vi "PRM - GetParameter.vi"(8 "error in (no error)":errorcluster, 11 "PRM":T1) -> (0 "error out":errorcluster, 3 "PRM OUT":T1, 5 "ParameterString":string)   [LabVIEW 2015]
doc: "Low Level function call. Converts LabVIEW enumeration to xiAPI parameter String."
uses:
  C:/GIT/Cameras3.x/Integrations/Labview/xiLib/xiLIB_32bit/xiLIB/xiCamLib/API/x86/xiApi.NET.dll
  xiLIB_32bit/xiLIB/xiCamLib/API/x86/xiApi.NET.dll
  PRM_v2.ctl
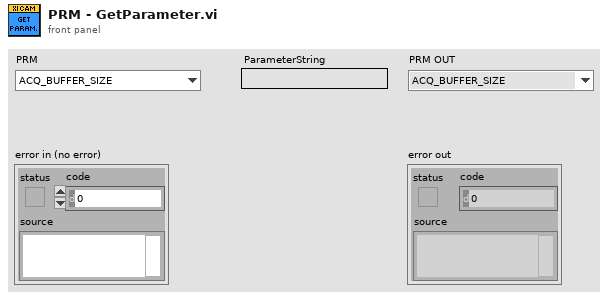
[diagram p1: front panel]
types:
  T1 = typedef "PRM_v2.ctl" = enum16{"ACQ_BUFFER_SIZE", "ACQ_FRAME_BURST_COUNT", "ACQ_TIMING_MODE", "ACQ_TRANSPORT_BUFFER_SIZE", "AE_MAX_LIMIT", "AEAG", "AEAG_LEVEL", "API_VERSION", "AG_MAX_LIMIT", "APPLY_CMS", "AUTO_BANDWIDTH_CALCULATION", "AUTO_WB", "AVAILABLE_BANDWIDTH", "AVAILABLE_BANDWIDTH_MAX", "AVAILABLE_BANDWIDTH_MIN", "BPC", "BUFFER_POLICY", "BUFFERS_QUEUE_SIZE", "CC_MATRIX_00", "CC_MATRIX_01", "CC_MATRIX_02", "CC_MATRIX_03", "CC_MATRIX_10", "CC_MATRIX_11", "CC_MATRIX_12", "CC_MATRIX_13", "CC_MATRIX_20", "CC_MATRIX_21", "CC_MATRIX_22", "CC_MATRIX_23", "CC_MATRIX_30", "CC_MATRIX_31", "CC_MATRIX_32", "CC_MATRIX_33", "CHIP_TEMP", "CMS", "COLOR_FILTER_ARRAY", "COOLING", "DEBOUNCE_EN", "DEBOUNCE_POL", "DEBOUNCE_T0", "DEBOUNCE_T1", "DEBUG_LEVEL", "DEFAULT_CC_MATRIX", "DEVICE_INSTANCE_PATH", "DEVICE_MODEL_ID", "DEVICE_NAME", "DEVICE_SN", "DEVICE_TYPE", "DEVICE_USER_ID", "DOWNSAMPLING", "DOWNSAMPLING_MAX", "DOWNSAMPLING_MIN", "DOWNSAMPLING_TYPE", "DRV_VERSION", "EXP_PRIORITY", "EXPOSURE", "EXPOSURE_DIRECT_UPDATE", "EXPOSURE_MAX", "EXPOSURE_MIN", "FFS_FILE_NAME", "FPGA1_VERSION", "FRAMERATE", "FRAMERATE_MAX", "FRAMERATE_MIN", "FREE_FFS_SIZE", "GAIN", "GAIN_DIRECT_UPDATE", "GAIN_MAX", "GAIN_MIN", "GAMMAC", "GAMMAY", "GPI_LEVEL", "GPI_MODE", "GPI_SELECTOR", "GPI_SELECTOR_MAX", "GPI_SELECTOR_MIN", "GPO_MODE", "GPO_SELECTOR", "GPO_SELECTOR_MAX", "GPO_SELECTOR_MIN", "HDR", "HDR_T1", "HDR_T2", "HEIGHT", "HEIGHT_MAX", "HEIGHT_MIN", "HOUSE_TEMP", "IMAGE_DATA_FORMAT", "IMAGE_IS_COLOR", "INPUT_CMS_PROFILE", "IS_COOLED", "IS_DEVICE_EXIST", "KNEEPOINT1", "KNEEPOINT2", "LED_MODE", "LED_SELECTOR", "LED_SELECTOR_MAX", "LED_SELECTOR_MIN", "LIMIT_BANDWIDTH", "LIMIT_BANDWIDTH_MAX", "LIMIT_BANDWIDTH_MIN", "LUT_EN", "LUT_INDEX", "LUT_INDEX_MAX", "LUT_INDEX_MIN", "LUT_VALUE", "LUT_VALUE_MAX", "LUT_VALUE_MIN", "MANUAL_WB", "MCU1_VERSION", "MCU2_VERSION", "OFFSET_X", "OFFSET_X_MAX", "OFFSET_X_MIN", "OFFSET_Y", "OFFSET_Y_MAX", "OFFSET_Y_MIN", "OUTPUT_CMS_PROFILE", "OUTPUT_DATA_BIT_DEPTH", "OUTPUT_DATA_PACKING", "READ_FILE_FFS", "RECENT_FRAME", "SENSOR_DATA_BIT_DEPTH", "SENSOR_MODE", "SENSOR_TAPS", "SHARPNESS", "SHUTTER_TYPE", "TARGET_TEMP", "TRG_DELAY", "TRG_SELECTOR", "TRG_SOFTWARE", "TRG_SOURCE", "USED_FFS_SIZE", "WB_KB", "WB_KG", "WB_KR", "WIDTH", "WIDTH_MAX", "WIDTH_MIN", "WRITE_FILE_FFS", "ACQ_BUFFER_SIZE_UNIT", "ACQ_TRANSPORT_BUFFER_COMMIT", "AEAG_ROI_HEIGHT", "AEAG_ROI_OFFSET_X", "AEAG_ROU_OFFSET_Y", "AEAG_ROI_WIDTH", "API_CONTEXT_LIST", "BINNING_HORIZONTAL", "BINNING_SELECTOR", "BINNING_VERTICAL", "COLUMN_FPN_CORRECTION", "COUNTER_SELECTOR", "COUNTER_VALUE", "DECIMATION_HORIZONTAL", "DECIMATION_SELECTOR", "DECIMATION_VERTICAL", "DEVICE_ID", "DEVICE_LOCATION_PATH", "DEVICE_MANIFEST", "DEVICE_RESET", "DEVICE_SENS_SN", "EXPOSURE_BURST_COUNT", "FFS_ACCESS_KEY", "GAIN_SELECTOR", "HW_REVISION", "IMAGE_BLACK_LEVEL", "IMAGE_DATA_BIT_DEPTH", "IMAGE_DATA_FORMAT_RGB32_ALPHA", "IMAGE_PAYLOAD_SIZE", "LENS_APERTURE_VALUE", "LENS_FEATURE", "LENS_FEATURE_SELECTOR", "LENS_FOCAL_LENGTH", "LENS_FOCUS_DISTANCE", "LENS_FOCUS_MOVE", "LENS_FOCUS_MOVEMENT_VALUE", "LENS_MODE", "OUTPUT_DATA_PACKING_TYPE", "SENSOR_CLOCK_FREQ_HZ", "SENSOR_CLOCK_FREQ_INDEX", "SENSOR_FEATURE_SELECTOR", "SENSOR_FEATURE_VALUE", "SENSOR_OUTPUT_CHANNEL_COUNT", "TRANSPORT_PIXEL_FORMAT", "TS_RST_MODE", "TS_RST_SOURCE"}
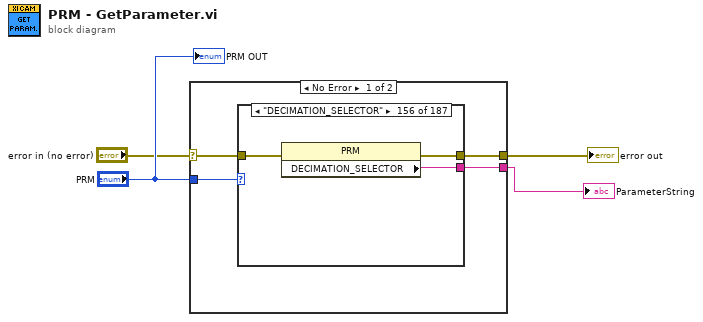
[diagram p0: block diagram]
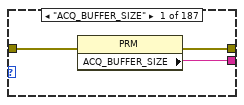
[diagram p2: hidden frame]
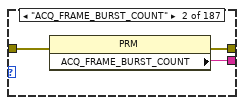
[diagram p3: hidden frame]
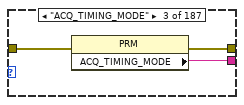
[diagram p4: hidden frame]
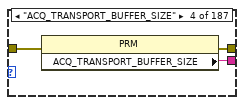
[diagram p5: hidden frame]
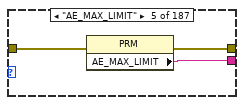
[diagram p6: hidden frame]
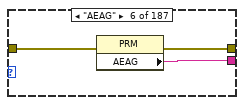
[diagram p7: hidden frame]
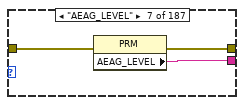
[diagram p8: hidden frame]
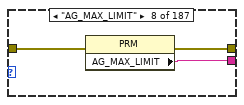
[diagram p9: hidden frame]
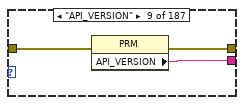
[diagram p10: hidden frame]
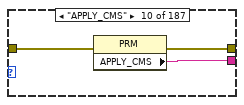
[diagram p11: hidden frame]
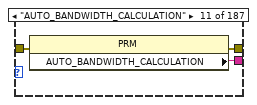
[diagram p12: hidden frame]
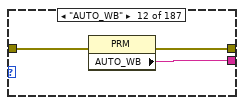
[diagram p13: hidden frame]
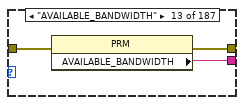
[diagram p14: hidden frame]
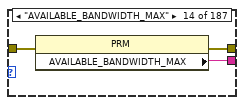
[diagram p15: hidden frame]
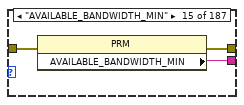
[diagram p16: hidden frame]
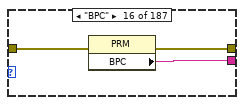
[diagram p17: hidden frame]
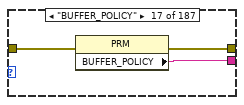
[diagram p18: hidden frame]
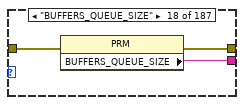
[diagram p19: hidden frame]
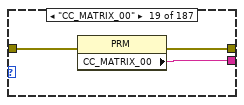
[diagram p20: hidden frame]
diagram:
  n1 = case shown="No Error" "error in (no error)" {
    selector: "error in (no error)" -> [w7 w570]
    tunnel: "PRM" -> [w8 _]
    tunnel: [w6 _] -> w1
    tunnel: [w5 w570] -> w2
    frame No Error {
      n2 = case shown="\"DECIMATION_SELECTOR\"" w8 {
        tunnel: w7 -> [w11 w14 w17 w20 w23 w26 w29 w32 w35 w38 w41 w44 w47 w50 w53 w56 w59 w62 w65 w68 w71 w74 w77 w80 w83 w86 w89 w92 w95 w98 w101 w104 w107 w110 w113 w116 w119 w122 w125 w128 w131 w134 w137 w140 w143 w146 w149 w152 w155 w158 w161 w164 w167 w170 w173 w176 w179 w182 w185 w188 w191 w194 w197 w200 w203 w206 w209 w212 w215 w218 w221 w224 w227 w230 w233 w236 w239 w242 w245 w248 w251 w254 w257 w260 w263 w266 w269 w272 w275 w278 w281 w284 w287 w290 w293 w296 w299 w302 w305 w308 w311 w314 w317 w320 w323 w326 w329 w332 w335 w338 w341 w344 w347 w350 w353 w356 w359 w362 w365 w368 w371 w374 w377 w380 w383 w386 w389 w392 w395 w398 w401 w404 w407 w410 w413 w416 w419 w422 w425 w428 w431 w434 w437 w440 w443 w446 w449 w452 w455 w458 w461 w464 w467 w470 w473 w476 w479 w482 w485 w488 w491 w494 w497 w500 w503 w506 w509 w512 w515 w518 w521 w524 w527 w530 w533 w536 w539 w542 w545 w548 w551 w554 w557 w560 w563 w566 w569]
        tunnel: [w10 w13 w16 w19 w22 w25 w28 w31 w34 w37 w40 w43 w46 w49 w52 w55 w58 w61 w64 w67 w70 w73 w76 w79 w82 w85 w88 w91 w94 w97 w100 w103 w106 w109 w112 w115 w118 w121 w124 w127 w130 w133 w136 w139 w142 w145 w148 w151 w154 w157 w160 w163 w166 w169 w172 w175 w178 w181 w184 w187 w190 w193 w196 w199 w202 w205 w208 w211 w214 w217 w220 w223 w226 w229 w232 w235 w238 w241 w244 w247 w250 w253 w256 w259 w262 w265 w268 w271 w274 w277 w280 w283 w286 w289 w292 w295 w298 w301 w304 w307 w310 w313 w316 w319 w322 w325 w328 w331 w334 w337 w340 w343 w346 w349 w352 w355 w358 w361 w364 w367 w370 w373 w376 w379 w382 w385 w388 w391 w394 w397 w400 w403 w406 w409 w412 w415 w418 w421 w424 w427 w430 w433 w436 w439 w442 w445 w448 w451 w454 w457 w460 w463 w466 w469 w472 w475 w478 w481 w484 w487 w490 w493 w496 w499 w502 w505 w508 w511 w514 w517 w520 w523 w526 w529 w532 w535 w538 w541 w544 w547 w550 w553 w556 w559 w562 w565 w568] -> w6
        tunnel: [w9 w12 w15 w18 w21 w24 w27 w30 w33 w36 w39 w42 w45 w48 w51 w54 w57 w60 w63 w66 w69 w72 w75 w78 w81 w84 w87 w90 w93 w96 w99 w102 w105 w108 w111 w114 w117 w120 w123 w126 w129 w132 w135 w138 w141 w144 w147 w150 w153 w156 w159 w162 w165 w168 w171 w174 w177 w180 w183 w186 w189 w192 w195 w198 w201 w204 w207 w210 w213 w216 w219 w222 w225 w228 w231 w234 w237 w240 w243 w246 w249 w252 w255 w258 w261 w264 w267 w270 w273 w276 w279 w282 w285 w288 w291 w294 w297 w300 w303 w306 w309 w312 w315 w318 w321 w324 w327 w330 w333 w336 w339 w342 w345 w348 w351 w354 w357 w360 w363 w366 w369 w372 w375 w378 w381 w384 w387 w390 w393 w396 w399 w402 w405 w408 w411 w414 w417 w420 w423 w426 w429 w432 w435 w438 w441 w444 w447 w450 w453 w456 w459 w462 w465 w468 w471 w474 w477 w480 w483 w486 w489 w492 w495 w498 w501 w504 w507 w510 w513 w516 w519 w522 w525 w528 w531 w534 w537 w540 w543 w546 w549 w552 w555 w558 w561 w564 w567] -> w5
        frame "ACQ_BUFFER_SIZE" {
          n3 = property class="PRM"(error in=w11) -> (error out=w9:errorcluster, "ACQ_BUFFER_SIZE"=w10:string)  [unwired: 1 in, 1 out]
        }
        frame "ACQ_FRAME_BURST_COUNT" {
          n4 = property class="PRM"(error in=w14) -> (error out=w12:errorcluster, "ACQ_FRAME_BURST_COUNT"=w13:string)  [unwired: 1 in, 1 out]
        }
        frame "ACQ_TIMING_MODE" {
          n5 = property class="PRM"(error in=w17) -> (error out=w15:errorcluster, "ACQ_TIMING_MODE"=w16:string)  [unwired: 1 in, 1 out]
        }
        frame "ACQ_TRANSPORT_BUFFER_SIZE" {
          n6 = property class="PRM"(error in=w20) -> (error out=w18:errorcluster, "ACQ_TRANSPORT_BUFFER_SIZE"=w19:string)  [unwired: 1 in, 1 out]
        }
        frame "AE_MAX_LIMIT" {
          n7 = property class="PRM"(error in=w23) -> (error out=w21:errorcluster, "AE_MAX_LIMIT"=w22:string)  [unwired: 1 in, 1 out]
        }
        frame "AEAG" {
          n8 = property class="PRM"(error in=w26) -> (error out=w24:errorcluster, "AEAG"=w25:string)  [unwired: 1 in, 1 out]
        }
        frame "AEAG_LEVEL" {
          n9 = property class="PRM"(error in=w29) -> (error out=w27:errorcluster, "AEAG_LEVEL"=w28:string)  [unwired: 1 in, 1 out]
        }
        frame "AG_MAX_LIMIT" {
          n10 = property class="PRM"(error in=w32) -> (error out=w30:errorcluster, "AG_MAX_LIMIT"=w31:string)  [unwired: 1 in, 1 out]
        }
        frame "API_VERSION" {
          n11 = property class="PRM"(error in=w35) -> (error out=w33:errorcluster, "API_VERSION"=w34:string)  [unwired: 1 in, 1 out]
        }
        frame "APPLY_CMS" {
          n12 = property class="PRM"(error in=w38) -> (error out=w36:errorcluster, "APPLY_CMS"=w37:string)  [unwired: 1 in, 1 out]
        }
        frame "AUTO_BANDWIDTH_CALCULATION" {
          n13 = property class="PRM"(error in=w41) -> (error out=w39:errorcluster, "AUTO_BANDWIDTH_CALCULATION"=w40:string)  [unwired: 1 in, 1 out]
        }
        frame "AUTO_WB" {
          n14 = property class="PRM"(error in=w44) -> (error out=w42:errorcluster, "AUTO_WB"=w43:string)  [unwired: 1 in, 1 out]
        }
        frame "AVAILABLE_BANDWIDTH" {
          n15 = property class="PRM"(error in=w47) -> (error out=w45:errorcluster, "AVAILABLE_BANDWIDTH"=w46:string)  [unwired: 1 in, 1 out]
        }
        frame "AVAILABLE_BANDWIDTH_MAX" {
          n16 = property class="PRM"(error in=w50) -> (error out=w48:errorcluster, "AVAILABLE_BANDWIDTH_MAX"=w49:string)  [unwired: 1 in, 1 out]
        }
        frame "AVAILABLE_BANDWIDTH_MIN" {
          n17 = property class="PRM"(error in=w53) -> (error out=w51:errorcluster, "AVAILABLE_BANDWIDTH_MIN"=w52:string)  [unwired: 1 in, 1 out]
        }
        frame "BPC" {
          n18 = property class="PRM"(error in=w56) -> (error out=w54:errorcluster, "BPC"=w55:string)  [unwired: 1 in, 1 out]
        }
        frame "BUFFER_POLICY" {
          n19 = property class="PRM"(error in=w59) -> (error out=w57:errorcluster, "BUFFER_POLICY"=w58:string)  [unwired: 1 in, 1 out]
        }
        frame "BUFFERS_QUEUE_SIZE" {
          n20 = property class="PRM"(error in=w62) -> (error out=w60:errorcluster, "BUFFERS_QUEUE_SIZE"=w61:string)  [unwired: 1 in, 1 out]
        }
        frame "CC_MATRIX_00" {
          n21 = property class="PRM"(error in=w65) -> (error out=w63:errorcluster, "CC_MATRIX_00"=w64:string)  [unwired: 1 in, 1 out]
        }
        frame "CC_MATRIX_01" {
          n22 = property class="PRM"(error in=w68) -> (error out=w66:errorcluster, "CC_MATRIX_01"=w67:string)  [unwired: 1 in, 1 out]
        }
        frame "CC_MATRIX_02" {
          n23 = property class="PRM"(error in=w71) -> (error out=w69:errorcluster, "CC_MATRIX_02"=w70:string)  [unwired: 1 in, 1 out]
        }
        frame "CC_MATRIX_03" {
          n24 = property class="PRM"(error in=w74) -> (error out=w72:errorcluster, "CC_MATRIX_03"=w73:string)  [unwired: 1 in, 1 out]
        }
        frame "CC_MATRIX_10" {
          n25 = property class="PRM"(error in=w77) -> (error out=w75:errorcluster, "CC_MATRIX_10"=w76:string)  [unwired: 1 in, 1 out]
        }
        frame "CC_MATRIX_11" {
          n26 = property class="PRM"(error in=w80) -> (error out=w78:errorcluster, "CC_MATRIX_11"=w79:string)  [unwired: 1 in, 1 out]
        }
        frame "CC_MATRIX_12" {
          n27 = property class="PRM"(error in=w83) -> (error out=w81:errorcluster, "CC_MATRIX_12"=w82:string)  [unwired: 1 in, 1 out]
        }
        frame "CC_MATRIX_13" {
          n28 = property class="PRM"(error in=w86) -> (error out=w84:errorcluster, "CC_MATRIX_13"=w85:string)  [unwired: 1 in, 1 out]
        }
        frame "CC_MATRIX_20" {
          n29 = property class="PRM"(error in=w89) -> (error out=w87:errorcluster, "CC_MATRIX_20"=w88:string)  [unwired: 1 in, 1 out]
        }
        frame "CC_MATRIX_21" {
          n30 = property class="PRM"(error in=w92) -> (error out=w90:errorcluster, "CC_MATRIX_21"=w91:string)  [unwired: 1 in, 1 out]
        }
        frame "CC_MATRIX_22" {
          n31 = property class="PRM"(error in=w95) -> (error out=w93:errorcluster, "CC_MATRIX_22"=w94:string)  [unwired: 1 in, 1 out]
        }
        frame "CC_MATRIX_23" {
          n32 = property class="PRM"(error in=w98) -> (error out=w96:errorcluster, "CC_MATRIX_23"=w97:string)  [unwired: 1 in, 1 out]
        }
        frame "CC_MATRIX_30" {
          n33 = property class="PRM"(error in=w101) -> (error out=w99:errorcluster, "CC_MATRIX_30"=w100:string)  [unwired: 1 in, 1 out]
        }
        frame "CC_MATRIX_31" {
          n34 = property class="PRM"(error in=w104) -> (error out=w102:errorcluster, "CC_MATRIX_31"=w103:string)  [unwired: 1 in, 1 out]
        }
        frame "CC_MATRIX_32" {
          n35 = property class="PRM"(error in=w107) -> (error out=w105:errorcluster, "CC_MATRIX_32"=w106:string)  [unwired: 1 in, 1 out]
        }
        frame "CC_MATRIX_33" {
          n36 = property class="PRM"(error in=w110) -> (error out=w108:errorcluster, "CC_MATRIX_33"=w109:string)  [unwired: 1 in, 1 out]
        }
        frame "CHIP_TEMP" {
          n37 = property class="PRM"(error in=w113) -> (error out=w111:errorcluster, "CHIP_TEMP"=w112:string)  [unwired: 1 in, 1 out]
        }
        frame "CMS" {
          n38 = property class="PRM"(error in=w116) -> (error out=w114:errorcluster, "CMS"=w115:string)  [unwired: 1 in, 1 out]
        }
        frame "COLOR_FILTER_ARRAY" {
          n39 = property class="PRM"(error in=w119) -> (error out=w117:errorcluster, "COLOR_FILTER_ARRAY"=w118:string)  [unwired: 1 in, 1 out]
        }
        frame "COOLING" {
          n40 = property class="PRM"(error in=w122) -> (error out=w120:errorcluster, "COOLING"=w121:string)  [unwired: 1 in, 1 out]
        }
        frame "DEBOUNCE_EN" {
          n41 = property class="PRM"(error in=w125) -> (error out=w123:errorcluster, "DEBOUNCE_EN"=w124:string)  [unwired: 1 in, 1 out]
        }
        frame "DEBOUNCE_POL" {
          n42 = property class="PRM"(error in=w128) -> (error out=w126:errorcluster, "DEBOUNCE_POL"=w127:string)  [unwired: 1 in, 1 out]
        }
        frame "DEBOUNCE_T0" {
          n43 = property class="PRM"(error in=w131) -> (error out=w129:errorcluster, "DEBOUNCE_T0"=w130:string)  [unwired: 1 in, 1 out]
        }
        frame "DEBOUNCE_T1" {
          n44 = property class="PRM"(error in=w134) -> (error out=w132:errorcluster, "DEBOUNCE_T1"=w133:string)  [unwired: 1 in, 1 out]
        }
        frame "DEBUG_LEVEL" {
          n45 = property class="PRM"(error in=w137) -> (error out=w135:errorcluster, "DEBUG_LEVEL"=w136:string)  [unwired: 1 in, 1 out]
        }
        frame "DEFAULT_CC_MATRIX" {
          n46 = property class="PRM"(error in=w140) -> (error out=w138:errorcluster, "DEFAULT_CC_MATRIX"=w139:string)  [unwired: 1 in, 1 out]
        }
        frame "DEVICE_INSTANCE_PATH" {
          n47 = property class="PRM"(error in=w143) -> (error out=w141:errorcluster, "DEVICE_INSTANCE_PATH"=w142:string)  [unwired: 1 in, 1 out]
        }
        frame "DEVICE_MODEL_ID" {
          n48 = property class="PRM"(error in=w146) -> (error out=w144:errorcluster, "DEVICE_MODEL_ID"=w145:string)  [unwired: 1 in, 1 out]
        }
        frame "DEVICE_NAME" {
          n49 = property class="PRM"(error in=w149) -> (error out=w147:errorcluster, "DEVICE_NAME"=w148:string)  [unwired: 1 in, 1 out]
        }
        frame "DEVICE_SN" {
          n50 = property class="PRM"(error in=w152) -> (error out=w150:errorcluster, "DEVICE_SN"=w151:string)  [unwired: 1 in, 1 out]
        }
        frame "DEVICE_TYPE" {
          n51 = property class="PRM"(error in=w155) -> (error out=w153:errorcluster, "DEVICE_TYPE"=w154:string)  [unwired: 1 in, 1 out]
        }
        frame "DEVICE_USER_ID" {
          n52 = property class="PRM"(error in=w158) -> (error out=w156:errorcluster, "DEVICE_USER_ID"=w157:string)  [unwired: 1 in, 1 out]
        }
        frame "DOWNSAMPLING" {
          n53 = property class="PRM"(error in=w161) -> (error out=w159:errorcluster, "DOWNSAMPLING"=w160:string)  [unwired: 1 in, 1 out]
        }
        frame "DOWNSAMPLING_MAX" {
          n54 = property class="PRM"(error in=w164) -> (error out=w162:errorcluster, "DOWNSAMPLING_MAX"=w163:string)  [unwired: 1 in, 1 out]
        }
        frame "DOWNSAMPLING_MIN" {
          n55 = property class="PRM"(error in=w167) -> (error out=w165:errorcluster, "DOWNSAMPLING_MIN"=w166:string)  [unwired: 1 in, 1 out]
        }
        frame "DOWNSAMPLING_TYPE" {
          n56 = property class="PRM"(error in=w170) -> (error out=w168:errorcluster, "DOWNSAMPLING_TYPE"=w169:string)  [unwired: 1 in, 1 out]
        }
        frame "DRV_VERSION" {
          n57 = property class="PRM"(error in=w173) -> (error out=w171:errorcluster, "DRV_VERSION"=w172:string)  [unwired: 1 in, 1 out]
        }
        frame "EXP_PRIORITY" {
          n58 = property class="PRM"(error in=w176) -> (error out=w174:errorcluster, "EXP_PRIORITY"=w175:string)  [unwired: 1 in, 1 out]
        }
        frame "EXPOSURE" {
          n59 = property class="PRM"(error in=w179) -> (error out=w177:errorcluster, "EXPOSURE"=w178:string)  [unwired: 1 in, 1 out]
        }
        frame "EXPOSURE_DIRECT_UPDATE" {
          n60 = property class="PRM"(error in=w182) -> (error out=w180:errorcluster, "EXPOSURE_DIRECT_UPDATE"=w181:string)  [unwired: 1 in, 1 out]
        }
        frame "EXPOSURE_MAX" {
          n61 = property class="PRM"(error in=w185) -> (error out=w183:errorcluster, "EXPOSURE_MAX"=w184:string)  [unwired: 1 in, 1 out]
        }
        frame "EXPOSURE_MIN" {
          n62 = property class="PRM"(error in=w188) -> (error out=w186:errorcluster, "EXPOSURE_MIN"=w187:string)  [unwired: 1 in, 1 out]
        }
        frame "FFS_FILE_NAME" {
          n63 = property class="PRM"(error in=w191) -> (error out=w189:errorcluster, "FFS_FILE_NAME"=w190:string)  [unwired: 1 in, 1 out]
        }
        frame "FPGA1_VERSION" {
          n64 = property class="PRM"(error in=w194) -> (error out=w192:errorcluster, "FPGA1_VERSION"=w193:string)  [unwired: 1 in, 1 out]
        }
        frame "FRAMERATE" {
          n65 = property class="PRM"(error in=w197) -> (error out=w195:errorcluster, "FRAMERATE"=w196:string)  [unwired: 1 in, 1 out]
        }
        frame "FRAMERATE_MAX" {
          n66 = property class="PRM"(error in=w200) -> (error out=w198:errorcluster, "FRAMERATE_MAX"=w199:string)  [unwired: 1 in, 1 out]
        }
        frame "FRAMERATE_MIN" {
          n67 = property class="PRM"(error in=w203) -> (error out=w201:errorcluster, "FRAMERATE_MIN"=w202:string)  [unwired: 1 in, 1 out]
        }
        frame "FREE_FFS_SIZE" {
          n68 = property class="PRM"(error in=w206) -> (error out=w204:errorcluster, "FREE_FFS_SIZE"=w205:string)  [unwired: 1 in, 1 out]
        }
        frame "GAIN" {
          n69 = property class="PRM"(error in=w209) -> (error out=w207:errorcluster, "GAIN"=w208:string)  [unwired: 1 in, 1 out]
        }
        frame "GAIN_DIRECT_UPDATE" {
          n70 = property class="PRM"(error in=w212) -> (error out=w210:errorcluster, "GAIN_DIRECT_UPDATE"=w211:string)  [unwired: 1 in, 1 out]
        }
        frame "GAIN_MAX" {
          n71 = property class="PRM"(error in=w215) -> (error out=w213:errorcluster, "GAIN_MAX"=w214:string)  [unwired: 1 in, 1 out]
        }
        frame "GAIN_MIN" {
          n72 = property class="PRM"(error in=w218) -> (error out=w216:errorcluster, "GAIN_MIN"=w217:string)  [unwired: 1 in, 1 out]
        }
        frame "GAMMAC" {
          n73 = property class="PRM"(error in=w221) -> (error out=w219:errorcluster, "GAMMAC"=w220:string)  [unwired: 1 in, 1 out]
        }
        frame "GAMMAY" {
          n74 = property class="PRM"(error in=w224) -> (error out=w222:errorcluster, "GAMMAY"=w223:string)  [unwired: 1 in, 1 out]
        }
        frame "GPI_LEVEL" {
          n75 = property class="PRM"(error in=w227) -> (error out=w225:errorcluster, "GPI_LEVEL"=w226:string)  [unwired: 1 in, 1 out]
        }
        frame "GPI_MODE" {
          n76 = property class="PRM"(error in=w230) -> (error out=w228:errorcluster, "GPI_MODE"=w229:string)  [unwired: 1 in, 1 out]
        }
        frame "GPI_SELECTOR" {
          n77 = property class="PRM"(error in=w233) -> (error out=w231:errorcluster, "GPI_SELECTOR"=w232:string)  [unwired: 1 in, 1 out]
        }
        frame "GPI_SELECTOR_MAX" {
          n78 = property class="PRM"(error in=w236) -> (error out=w234:errorcluster, "GPI_SELECTOR_MAX"=w235:string)  [unwired: 1 in, 1 out]
        }
        frame "GPI_SELECTOR_MIN" {
          n79 = property class="PRM"(error in=w239) -> (error out=w237:errorcluster, "GPI_SELECTOR_MIN"=w238:string)  [unwired: 1 in, 1 out]
        }
        frame "GPO_MODE" {
          n80 = property class="PRM"(error in=w242) -> (error out=w240:errorcluster, "GPO_MODE"=w241:string)  [unwired: 1 in, 1 out]
        }
        frame "GPO_SELECTOR" {
          n81 = property class="PRM"(error in=w245) -> (error out=w243:errorcluster, "GPO_SELECTOR"=w244:string)  [unwired: 1 in, 1 out]
        }
        frame "GPO_SELECTOR_MAX" {
          n82 = property class="PRM"(error in=w248) -> (error out=w246:errorcluster, "GPO_SELECTOR_MAX"=w247:string)  [unwired: 1 in, 1 out]
        }
        frame "GPO_SELECTOR_MIN" {
          n83 = property class="PRM"(error in=w251) -> (error out=w249:errorcluster, "GPO_SELECTOR_MIN"=w250:string)  [unwired: 1 in, 1 out]
        }
        frame "HDR" {
          n84 = property class="PRM"(error in=w254) -> (error out=w252:errorcluster, "HDR"=w253:string)  [unwired: 1 in, 1 out]
        }
        frame "HDR_T1" {
          n85 = property class="PRM"(error in=w257) -> (error out=w255:errorcluster, "HDR_T1"=w256:string)  [unwired: 1 in, 1 out]
        }
        frame "HDR_T2" {
          n86 = property class="PRM"(error in=w260) -> (error out=w258:errorcluster, "HDR_T2"=w259:string)  [unwired: 1 in, 1 out]
        }
        frame "HEIGHT" {
          n87 = property class="PRM"(error in=w263) -> (error out=w261:errorcluster, "HEIGHT"=w262:string)  [unwired: 1 in, 1 out]
        }
        frame "HEIGHT_MAX" {
          n88 = property class="PRM"(error in=w266) -> (error out=w264:errorcluster, "HEIGHT_MAX"=w265:string)  [unwired: 1 in, 1 out]
        }
        frame "HEIGHT_MIN" {
          n89 = property class="PRM"(error in=w269) -> (error out=w267:errorcluster, "HEIGHT_MIN"=w268:string)  [unwired: 1 in, 1 out]
        }
        frame "HOUSE_TEMP" {
          n90 = property class="PRM"(error in=w272) -> (error out=w270:errorcluster, "HOUS_TEMP"=w271:string)  [unwired: 1 in, 1 out]
        }
        frame "IMAGE_DATA_FORMAT" {
          n91 = property class="PRM"(error in=w275) -> (error out=w273:errorcluster, "IMAGE_DATA_FORMAT"=w274:string)  [unwired: 1 in, 1 out]
        }
        frame "IMAGE_IS_COLOR" {
          n92 = property class="PRM"(error in=w278) -> (error out=w276:errorcluster, "IMAGE_IS_COLOR"=w277:string)  [unwired: 1 in, 1 out]
        }
        frame "INPUT_CMS_PROFILE" {
          n93 = property class="PRM"(error in=w281) -> (error out=w279:errorcluster, "INPUT_CMS_PROFILE"=w280:string)  [unwired: 1 in, 1 out]
        }
        frame "IS_COOLED" {
          n94 = property class="PRM"(error in=w284) -> (error out=w282:errorcluster, "IS_COOLED"=w283:string)  [unwired: 1 in, 1 out]
        }
        frame "IS_DEVICE_EXIST" {
          n95 = property class="PRM"(error in=w287) -> (error out=w285:errorcluster, "IS_DEVICE_EXIST"=w286:string)  [unwired: 1 in, 1 out]
        }
        frame "KNEEPOINT1" {
          n96 = property class="PRM"(error in=w290) -> (error out=w288:errorcluster, "KNEEPOINT1"=w289:string)  [unwired: 1 in, 1 out]
        }
        frame "KNEEPOINT2" {
          n97 = property class="PRM"(error in=w293) -> (error out=w291:errorcluster, "KNEEPOINT2"=w292:string)  [unwired: 1 in, 1 out]
        }
        frame "LED_MODE" {
          n98 = property class="PRM"(error in=w296) -> (error out=w294:errorcluster, "LED_MODE"=w295:string)  [unwired: 1 in, 1 out]
        }
        frame "LED_SELECTOR" {
          n99 = property class="PRM"(error in=w299) -> (error out=w297:errorcluster, "LED_SELECTOR"=w298:string)  [unwired: 1 in, 1 out]
        }
        frame "LED_SELECTOR_MAX" {
          n100 = property class="PRM"(error in=w302) -> (error out=w300:errorcluster, "LED_SELECTOR_MAX"=w301:string)  [unwired: 1 in, 1 out]
        }
        frame "LED_SELECTOR_MIN" {
          n101 = property class="PRM"(error in=w305) -> (error out=w303:errorcluster, "LED_SELECTOR_MIN"=w304:string)  [unwired: 1 in, 1 out]
        }
        frame "LIMIT_BANDWIDTH" {
          n102 = property class="PRM"(error in=w308) -> (error out=w306:errorcluster, "LIMIT_BANDWIDTH"=w307:string)  [unwired: 1 in, 1 out]
        }
        frame "LIMIT_BANDWIDTH_MAX" {
          n103 = property class="PRM"(error in=w311) -> (error out=w309:errorcluster, "LIMIT_BANDWIDTH_MAX"=w310:string)  [unwired: 1 in, 1 out]
        }
        frame "LIMIT_BANDWIDTH_MIN" {
          n104 = property class="PRM"(error in=w314) -> (error out=w312:errorcluster, "LIMIT_BANDWIDTH_MIN"=w313:string)  [unwired: 1 in, 1 out]
        }
        frame "LUT_EN" {
          n105 = property class="PRM"(error in=w317) -> (error out=w315:errorcluster, "LUT_EN"=w316:string)  [unwired: 1 in, 1 out]
        }
        frame "LUT_INDEX" {
          n106 = property class="PRM"(error in=w320) -> (error out=w318:errorcluster, "LUT_INDEX"=w319:string)  [unwired: 1 in, 1 out]
        }
        frame "LUT_INDEX_MAX" {
          n107 = property class="PRM"(error in=w323) -> (error out=w321:errorcluster, "LUT_INDEX_MAX"=w322:string)  [unwired: 1 in, 1 out]
        }
        frame "LUT_INDEX_MIN" {
          n108 = property class="PRM"(error in=w326) -> (error out=w324:errorcluster, "LUT_INDEX_MIN"=w325:string)  [unwired: 1 in, 1 out]
        }
        frame "LUT_VALUE" {
          n109 = property class="PRM"(error in=w329) -> (error out=w327:errorcluster, "LUT_VALUE"=w328:string)  [unwired: 1 in, 1 out]
        }
        frame "LUT_VALUE_MAX" {
          n110 = property class="PRM"(error in=w332) -> (error out=w330:errorcluster, "LUT_VALUE_MAX"=w331:string)  [unwired: 1 in, 1 out]
        }
        frame "LUT_VALUE_MIN" {
          n111 = property class="PRM"(error in=w335) -> (error out=w333:errorcluster, "LUT_VALUE_MIN"=w334:string)  [unwired: 1 in, 1 out]
        }
        frame "MANUAL_WB" {
          n112 = property class="PRM"(error in=w338) -> (error out=w336:errorcluster, "MANUAL_WB"=w337:string)  [unwired: 1 in, 1 out]
        }
        frame "MCU1_VERSION" {
          n113 = property class="PRM"(error in=w341) -> (error out=w339:errorcluster, "MCU1_VERSION"=w340:string)  [unwired: 1 in, 1 out]
        }
        frame "MCU2_VERSION" {
          n114 = property class="PRM"(error in=w344) -> (error out=w342:errorcluster, "MCU2_VERSION"=w343:string)  [unwired: 1 in, 1 out]
        }
        frame "OFFSET_X" {
          n115 = property class="PRM"(error in=w347) -> (error out=w345:errorcluster, "OFFSET_X"=w346:string)  [unwired: 1 in, 1 out]
        }
        frame "OFFSET_X_MAX" {
          n116 = property class="PRM"(error in=w350) -> (error out=w348:errorcluster, "OFFSET_X_MAX"=w349:string)  [unwired: 1 in, 1 out]
        }
        frame "OFFSET_X_MIN" {
          n117 = property class="PRM"(error in=w353) -> (error out=w351:errorcluster, "OFFSET_X_MIN"=w352:string)  [unwired: 1 in, 1 out]
        }
        frame "OFFSET_Y" {
          n118 = property class="PRM"(error in=w356) -> (error out=w354:errorcluster, "OFFSET_Y"=w355:string)  [unwired: 1 in, 1 out]
        }
        frame "OFFSET_Y_MAX" {
          n119 = property class="PRM"(error in=w359) -> (error out=w357:errorcluster, "OFFSET_Y_MAX"=w358:string)  [unwired: 1 in, 1 out]
        }
        frame "OFFSET_Y_MIN" {
          n120 = property class="PRM"(error in=w362) -> (error out=w360:errorcluster, "OFFSET_Y_MIN"=w361:string)  [unwired: 1 in, 1 out]
        }
        frame "OUTPUT_CMS_PROFILE" {
          n121 = property class="PRM"(error in=w365) -> (error out=w363:errorcluster, "OUTPUT_CMS_PROFILE"=w364:string)  [unwired: 1 in, 1 out]
        }
        frame "OUTPUT_DATA_BIT_DEPTH" {
          n122 = property class="PRM"(error in=w368) -> (error out=w366:errorcluster, "OUTPUT_DATA_BIT_DEPTH"=w367:string)  [unwired: 1 in, 1 out]
        }
        frame "OUTPUT_DATA_PACKING" {
          n123 = property class="PRM"(error in=w371) -> (error out=w369:errorcluster, "OUTPUT_DATA_PACKING"=w370:string)  [unwired: 1 in, 1 out]
        }
        frame "READ_FILE_FFS" {
          n124 = property class="PRM"(error in=w374) -> (error out=w372:errorcluster, "READ_FILE_FFS"=w373:string)  [unwired: 1 in, 1 out]
        }
        frame "RECENT_FRAME" {
          n125 = property class="PRM"(error in=w377) -> (error out=w375:errorcluster, "RECENT_FRAME"=w376:string)  [unwired: 1 in, 1 out]
        }
        frame "SENSOR_DATA_BIT_DEPTH" {
          n126 = property class="PRM"(error in=w380) -> (error out=w378:errorcluster, "SENSOR_DATA_BIT_DEPTH"=w379:string)  [unwired: 1 in, 1 out]
        }
        frame "SENSOR_MODE" {
          n127 = property class="PRM"(error in=w383) -> (error out=w381:errorcluster, "SENSOR_MODE"=w382:string)  [unwired: 1 in, 1 out]
        }
        frame "SENSOR_TAPS" {
          n128 = property class="PRM"(error in=w386) -> (error out=w384:errorcluster, "SENSOR_TAPS"=w385:string)  [unwired: 1 in, 1 out]
        }
        frame "SHARPNESS" {
          n129 = property class="PRM"(error in=w389) -> (error out=w387:errorcluster, "SHARPNESS"=w388:string)  [unwired: 1 in, 1 out]
        }
        frame "SHUTTER_TYPE" {
          n130 = property class="PRM"(error in=w392) -> (error out=w390:errorcluster, "SHUTTER_TYPE"=w391:string)  [unwired: 1 in, 1 out]
        }
        frame "TARGET_TEMP" {
          n131 = property class="PRM"(error in=w395) -> (error out=w393:errorcluster, "TARGET_TEMP"=w394:string)  [unwired: 1 in, 1 out]
        }
        frame "TRG_DELAY" {
          n132 = property class="PRM"(error in=w398) -> (error out=w396:errorcluster, "TRG_DELAY"=w397:string)  [unwired: 1 in, 1 out]
        }
        frame "TRG_SELECTOR" {
          n133 = property class="PRM"(error in=w401) -> (error out=w399:errorcluster, "TRG_SELECTOR"=w400:string)  [unwired: 1 in, 1 out]
        }
        frame "TRG_SOFTWARE" {
          n134 = property class="PRM"(error in=w404) -> (error out=w402:errorcluster, "TRG_SOFTWARE"=w403:string)  [unwired: 1 in, 1 out]
        }
        frame "TRG_SOURCE" {
          n135 = property class="PRM"(error in=w407) -> (error out=w405:errorcluster, "TRG_SOURCE"=w406:string)  [unwired: 1 in, 1 out]
        }
        frame "USED_FFS_SIZE" {
          n136 = property class="PRM"(error in=w410) -> (error out=w408:errorcluster, "USED_FFS_SIZE"=w409:string)  [unwired: 1 in, 1 out]
        }
        frame "WB_KB" {
          n137 = property class="PRM"(error in=w413) -> (error out=w411:errorcluster, "WB_KB"=w412:string)  [unwired: 1 in, 1 out]
        }
        frame "WB_KG" {
          n138 = property class="PRM"(error in=w416) -> (error out=w414:errorcluster, "WB_KG"=w415:string)  [unwired: 1 in, 1 out]
        }
        frame "WB_KR" {
          n139 = property class="PRM"(error in=w419) -> (error out=w417:errorcluster, "WB_KR"=w418:string)  [unwired: 1 in, 1 out]
        }
        frame "WIDTH" {
          n140 = property class="PRM"(error in=w422) -> (error out=w420:errorcluster, "WIDTH"=w421:string)  [unwired: 1 in, 1 out]
        }
        frame "WIDTH_MAX" {
          n141 = property class="PRM"(error in=w425) -> (error out=w423:errorcluster, "WIDTH_MAX"=w424:string)  [unwired: 1 in, 1 out]
        }
        frame "WIDTH_MIN" {
          n142 = property class="PRM"(error in=w428) -> (error out=w426:errorcluster, "WIDTH_MIN"=w427:string)  [unwired: 1 in, 1 out]
        }
        frame "WRITE_FILE_FFS" {
          n143 = property class="PRM"(error in=w431) -> (error out=w429:errorcluster, "WRITE_FILE_FFS"=w430:string)  [unwired: 1 in, 1 out]
        }
        frame "ACQ_BUFFER_SIZE_UNIT" {
          n144 = property class="PRM"(error in=w434) -> (error out=w432:errorcluster, "ACQ_BUFFER_SIZE_UNIT"=w433:string)  [unwired: 1 in, 1 out]
        }
        frame "ACQ_TRANSPORT_BUFFER_COMMIT" {
          n145 = property class="PRM"(error in=w437) -> (error out=w435:errorcluster, "ACQ_TRANSPORT_BUFFER_COMMIT"=w436:string)  [unwired: 1 in, 1 out]
        }
        frame "AEAG_ROI_HEIGHT" {
          n146 = property class="PRM"(error in=w440) -> (error out=w438:errorcluster, "AEAG_ROI_HEIGHT"=w439:string)  [unwired: 1 in, 1 out]
        }
        frame "AEAG_ROI_OFFSET_X" {
          n147 = property class="PRM"(error in=w443) -> (error out=w441:errorcluster, "AEAG_ROI_OFFSET_X"=w442:string)  [unwired: 1 in, 1 out]
        }
        frame "AEAG_ROU_OFFSET_Y" {
          n148 = property class="PRM"(error in=w446) -> (error out=w444:errorcluster, "AEAG_ROI_OFFSET_Y"=w445:string)  [unwired: 1 in, 1 out]
        }
        frame "AEAG_ROI_WIDTH" {
          n149 = property class="PRM"(error in=w449) -> (error out=w447:errorcluster, "AEAG_ROI_WIDTH"=w448:string)  [unwired: 1 in, 1 out]
        }
        frame "API_CONTEXT_LIST" {
          n150 = property class="PRM"(error in=w452) -> (error out=w450:errorcluster, "API_CONTEXT_LIST"=w451:string)  [unwired: 1 in, 1 out]
        }
        frame "BINNING_HORIZONTAL" {
          n151 = property class="PRM"(error in=w455) -> (error out=w453:errorcluster, "BINNING_HORIZONTAL"=w454:string)  [unwired: 1 in, 1 out]
        }
        frame "BINNING_SELECTOR" {
          n152 = property class="PRM"(error in=w458) -> (error out=w456:errorcluster, "BINNING_SELECTOR"=w457:string)  [unwired: 1 in, 1 out]
        }
        frame "BINNING_VERTICAL" {
          n153 = property class="PRM"(error in=w461) -> (error out=w459:errorcluster, "BINNING_VERTICAL"=w460:string)  [unwired: 1 in, 1 out]
        }
        frame "COLUMN_FPN_CORRECTION" {
          n154 = property class="PRM"(error in=w464) -> (error out=w462:errorcluster, "COLUMN_FPN_CORRECTION"=w463:string)  [unwired: 1 in, 1 out]
        }
        frame "COUNTER_SELECTOR" {
          n155 = property class="PRM"(error in=w467) -> (error out=w465:errorcluster, "COUNTER_SELECTOR"=w466:string)  [unwired: 1 in, 1 out]
        }
        frame "COUNTER_VALUE" {
          n156 = property class="PRM"(error in=w470) -> (error out=w468:errorcluster, "COUNTER_VALUE"=w469:string)  [unwired: 1 in, 1 out]
        }
        frame "DECIMATION_HORIZONTAL" {
          n157 = property class="PRM"(error in=w473) -> (error out=w471:errorcluster, "DECIMATION_HORIZONTAL"=w472:string)  [unwired: 1 in, 1 out]
        }
        frame "DECIMATION_SELECTOR" {
          n158 = property class="PRM"(error in=w476) -> (error out=w474:errorcluster, "DECIMATION_SELECTOR"=w475:string)  [unwired: 1 in, 1 out]
        }
        frame "DECIMATION_VERTICAL" {
          n159 = property class="PRM"(error in=w479) -> (error out=w477:errorcluster, "DECIMATION_VERTICAL"=w478:string)  [unwired: 1 in, 1 out]
        }
        frame "DEVICE_ID" {
          n160 = property class="PRM"(error in=w482) -> (error out=w480:errorcluster, "DEVICE_ID"=w481:string)  [unwired: 1 in, 1 out]
        }
        frame "DEVICE_LOCATION_PATH" {
          n161 = property class="PRM"(error in=w485) -> (error out=w483:errorcluster, "DEVICE_LOCATION_PATH"=w484:string)  [unwired: 1 in, 1 out]
        }
        frame "DEVICE_MANIFEST" {
          n162 = property class="PRM"(error in=w488) -> (error out=w486:errorcluster, "DEVICE_MANIFEST"=w487:string)  [unwired: 1 in, 1 out]
        }
        frame "DEVICE_RESET" {
          n163 = property class="PRM"(error in=w491) -> (error out=w489:errorcluster, "DEVICE_RESET"=w490:string)  [unwired: 1 in, 1 out]
        }
        frame "DEVICE_SENS_SN" {
          n164 = property class="PRM"(error in=w494) -> (error out=w492:errorcluster, "DEVICE_SENS_SN"=w493:string)  [unwired: 1 in, 1 out]
        }
        frame "EXPOSURE_BURST_COUNT" {
          n165 = property class="PRM"(error in=w497) -> (error out=w495:errorcluster, "EXPOSURE_BURST_COUNT"=w496:string)  [unwired: 1 in, 1 out]
        }
        frame "FFS_ACCESS_KEY" {
          n166 = property class="PRM"(error in=w500) -> (error out=w498:errorcluster, "FFS_ACCESS_KEY"=w499:string)  [unwired: 1 in, 1 out]
        }
        frame "GAIN_SELECTOR" {
          n167 = property class="PRM"(error in=w503) -> (error out=w501:errorcluster, "GAIN_SELECTOR"=w502:string)  [unwired: 1 in, 1 out]
        }
        frame "HW_REVISION" {
          n168 = property class="PRM"(error in=w506) -> (error out=w504:errorcluster, "HW_REVISION"=w505:string)  [unwired: 1 in, 1 out]
        }
        frame "IMAGE_BLACK_LEVEL" {
          n169 = property class="PRM"(error in=w509) -> (error out=w507:errorcluster, "IMAGE_BLACK_LEVEL"=w508:string)  [unwired: 1 in, 1 out]
        }
        frame "IMAGE_DATA_BIT_DEPTH" {
          n170 = property class="PRM"(error in=w512) -> (error out=w510:errorcluster, "IMAGE_DATA_BIT_DEPTH"=w511:string)  [unwired: 1 in, 1 out]
        }
        frame "IMAGE_DATA_FORMAT_RGB32_ALPHA" {
          n171 = property class="PRM"(error in=w515) -> (error out=w513:errorcluster, "IMAGE_DATA_FORMAT_RGB32_ALPHA"=w514:string)  [unwired: 1 in, 1 out]
        }
        frame "IMAGE_PAYLOAD_SIZE" {
          n172 = property class="PRM"(error in=w518) -> (error out=w516:errorcluster, "IMAGE_PAYLOAD_SIZE"=w517:string)  [unwired: 1 in, 1 out]
        }
        frame "LENS_APERTURE_VALUE" {
          n173 = property class="PRM"(error in=w521) -> (error out=w519:errorcluster, "LENS_APERTURE_VALUE"=w520:string)  [unwired: 1 in, 1 out]
        }
        frame "LENS_FEATURE" {
          n174 = property class="PRM"(error in=w524) -> (error out=w522:errorcluster, "LENS_FEATURE"=w523:string)  [unwired: 1 in, 1 out]
        }
        frame "LENS_FEATURE_SELECTOR" {
          n175 = property class="PRM"(error in=w527) -> (error out=w525:errorcluster, "LENS_FEATURE_SELECTOR"=w526:string)  [unwired: 1 in, 1 out]
        }
        frame "LENS_FOCAL_LENGTH" {
          n176 = property class="PRM"(error in=w530) -> (error out=w528:errorcluster, "LENS_FOCAL_LENGTH"=w529:string)  [unwired: 1 in, 1 out]
        }
        frame "LENS_FOCUS_DISTANCE" {
          n177 = property class="PRM"(error in=w533) -> (error out=w531:errorcluster, "LENS_FOCUS_DISTANCE"=w532:string)  [unwired: 1 in, 1 out]
        }
        frame "LENS_FOCUS_MOVE" {
          n178 = property class="PRM"(error in=w536) -> (error out=w534:errorcluster, "LENS_FOCUS_MOVE"=w535:string)  [unwired: 1 in, 1 out]
        }
        frame "LENS_FOCUS_MOVEMENT_VALUE" {
          n179 = property class="PRM"(error in=w539) -> (error out=w537:errorcluster, "LENS_FOCUS_MOVEMENT_VALUE"=w538:string)  [unwired: 1 in, 1 out]
        }
        frame "LENS_MODE" {
          n180 = property class="PRM"(error in=w542) -> (error out=w540:errorcluster, "LENS_MODE"=w541:string)  [unwired: 1 in, 1 out]
        }
        frame "OUTPUT_DATA_PACKING_TYPE" {
          n181 = property class="PRM"(error in=w545) -> (error out=w543:errorcluster, "OUTPUT_DATA_PACKING_TYPE"=w544:string)  [unwired: 1 in, 1 out]
        }
        frame "SENSOR_CLOCK_FREQ_HZ" {
          n182 = property class="PRM"(error in=w548) -> (error out=w546:errorcluster, "SENSOR_CLOCK_FREQ_HZ"=w547:string)  [unwired: 1 in, 1 out]
        }
        frame "SENSOR_CLOCK_FREQ_INDEX" {
          n183 = property class="PRM"(error in=w551) -> (error out=w549:errorcluster, "SENSOR_CLOCK_FREQ_INDEX"=w550:string)  [unwired: 1 in, 1 out]
        }
        frame "SENSOR_FEATURE_SELECTOR" {
          n184 = property class="PRM"(error in=w554) -> (error out=w552:errorcluster, "SENSOR_FEATURE_SELECTOR"=w553:string)  [unwired: 1 in, 1 out]
        }
        frame "SENSOR_FEATURE_VALUE" {
          n185 = property class="PRM"(error in=w557) -> (error out=w555:errorcluster, "SENSOR_FEATURE_VALUE"=w556:string)  [unwired: 1 in, 1 out]
        }
        frame "SENSOR_OUTPUT_CHANNEL_COUNT" {
          n186 = property class="PRM"(error in=w560) -> (error out=w558:errorcluster, "SENSOR_OUTPUT_CHANNEL_COUNT"=w559:string)  [unwired: 1 in, 1 out]
        }
        frame "TRANSPORT_PIXEL_FORMAT" {
          n187 = property class="PRM"(error in=w563) -> (error out=w561:errorcluster, "TRANSPORT_PIXEL_FORMAT"=w562:string)  [unwired: 1 in, 1 out]
        }
        frame "TS_RST_MODE" {
          n188 = property class="PRM"(error in=w566) -> (error out=w564:errorcluster, "TS_RST_MODE"=w565:string)  [unwired: 1 in, 1 out]
        }
        frame "TS_RST_SOURCE" {
          n189 = property class="PRM"(error in=w569) -> (error out=w567:errorcluster, "TS_RST_SOURCE"=w568:string)  [unwired: 1 in, 1 out]
        }
      }
    }
    frame Error {
    }
  }
  "error out" <- w2
  "ParameterString" <- w1
  "PRM OUT" <- "PRM"
